vi "DCA Recalculate Values.vi"(5 "Colors":cluster{"Pass":u32, "Fail":u32, "Nop":u32}={"Pass"=6618880, "Fail"=16711680, "Nop"=16777226}, 6 "Attenuation Calculation":enum32{"Power", "Voltage"}(ring), 7 "Limit Status Ref":refnum<vi>, 8 "error in (no error)":errorcluster, 9 "Test Parameters In":T8={"Stimulus"={"Use Instrument"=FALSE, "Normalize"=FALSE, "Blank Screen"=FALSE, "Measurement Type"=enum."Diode", "Range"=enum."Auto", "Resolution"=enum."Auto"}, "Measurement"={"Topology"=enum."PI-Network", "Lock Topology"=FALSE, "ATTN Calc"=enum."Power", "Zo"=50.0}, "Limits"=[], "Normalization"={"Normalized?"=FALSE, "Rab Value"=0.0, "Rac Value"=0.0, "Rbc Value"=0.0}}, 10 "Topology":T6, 11 "Measurement Values":T7) -> (0 "error out":errorcluster, 1 "Test Parameters Out":T8={"Stimulus"={"Use Instrument"=FALSE, "Normalize"=FALSE, "Blank Screen"=FALSE, "Measurement Type"=enum."Diode", "Range"=enum."Auto", "Resolution"=enum."Auto"}, "Measurement"={"Topology"=enum."PI-Network", "Lock Topology"=FALSE, "ATTN Calc"=enum."Power", "Zo"=50.0}, "Limits"=[], "Normalization"={"Normalized?"=FALSE, "Rab Value"=0.0, "Rac Value"=0.0, "Rbc Value"=0.0}}, 2 "Passed?":bool, 3 "Measurement Values":T7, 4 "Limits and Passed?":cluster{"Limits":T1[], "Passed? Array":bool[]})   [LabVIEW 2011]
uses:
  TypeDefs/DCA Test Parameters.ctl
  TypeDefs/DCA Stimulus Parameters.ctl
  TypeDefs/DCA Measurement Cluster.ctl
  TypeDefs/DCA Topology.ctl
  TypeDefs/DCA Attenuation Calculation.ctl
  TypeDefs/DCA Limit.ctl
  TypeDefs/DCA Limit Quantity.ctl
  TypeDefs/DCA Limit Comparison.ctl
  TypeDefs/DCA Limit Operation.ctl
  Test Referential Limit.ctl
  TypeDefs/DCA Calibration State.ctl
  TypeDefs/DCA Measurement Values.ctl
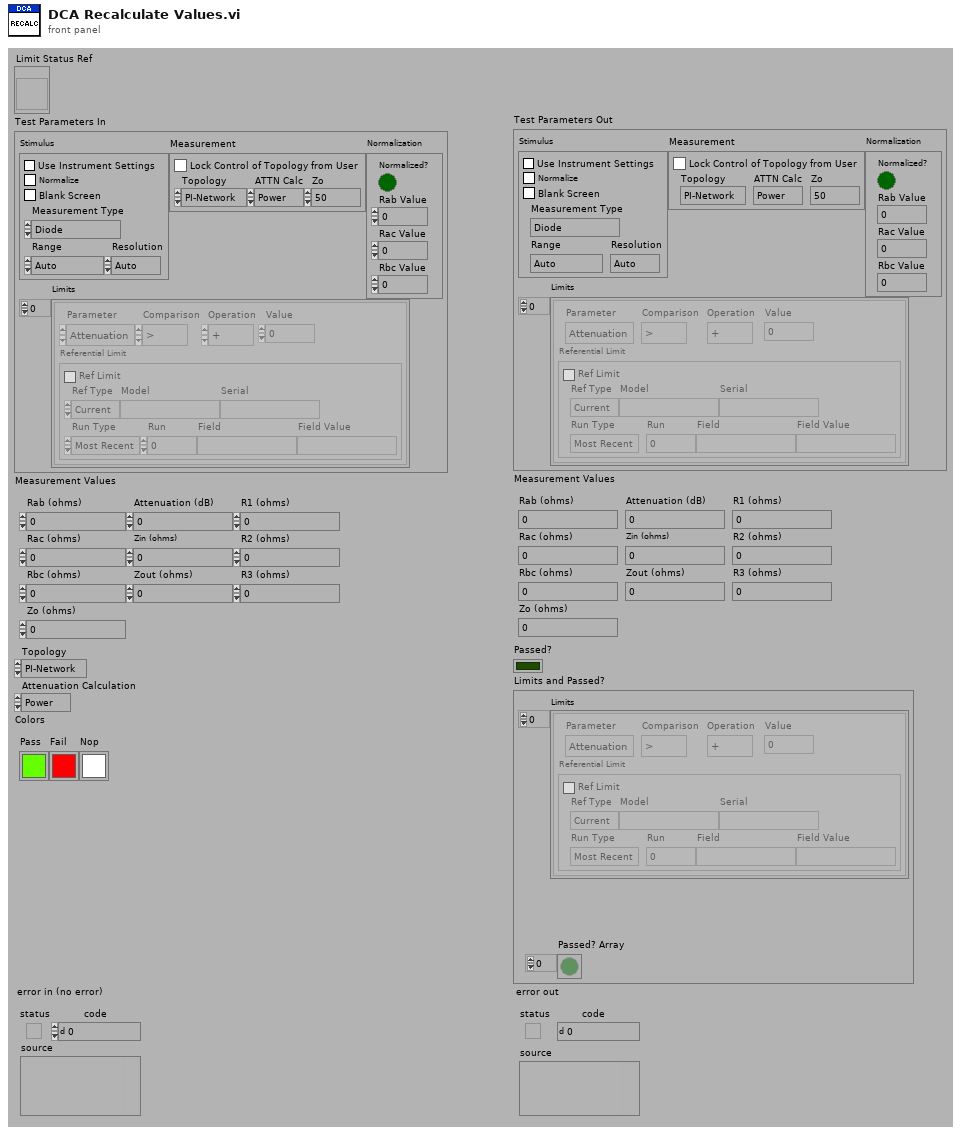
[diagram p1: front panel]
types:
  T1 = typedef "DCA Limit.ctl" = cluster{"Parameter":T2, "Comparison":T3, "Operation":T4, "Value":dbl, "Referential Limit":T5}
  T2 = typedef "DCA Limit Quantity.ctl" = enum16{"Attenuation", "Zin", "Zout", "R1", "R2", "R3", "Rab", "Rac", "Rbc"}
  T3 = typedef "DCA Limit Comparison.ctl" = enum16{">", ">=", "<", "<="}
  T4 = typedef "DCA Limit Operation.ctl" = enum16{"+", "-"}
  T5 = typedef "Test Referential Limit.ctl" = cluster{"Ref Limit":bool, "Ref Type":enum16{"Current", "Specify"}, "Model":string, "Serial":string, "Run Type":enum16{"Most Recent", "Run #", "Match Field"}, "Run":i32, "Field":string, "Field Value":string}
  T6 = typedef "DCA Topology.ctl" = enum32{"PI-Network", "T-Network"}
  T7 = typedef "DCA Measurement Values.ctl" = cluster{"Rab (ohms)":dbl, "Rac (ohms)":dbl, "Rbc (ohms)":dbl, "Zo (ohms)":dbl, "Attenuation (dB)":dbl, "Zin (ohms)":dbl, "Zout (ohms)":dbl, "R1 (ohms)":dbl, "R2 (ohms)":dbl, "R3 (ohms)":dbl}
  T8 = typedef "DCA Test Parameters.ctl" = cluster{"Stimulus":T9, "Measurement":T10, "Limits":T1[], "Normalization":T12}
  T9 = typedef "DCA Stimulus Parameters.ctl" = cluster{"Use Instrument":bool, "Normalize":bool, "Blank Screen":bool, "Measurement Type":enum16{"Voltage DC", "Voltage DC Ratio", "Voltage AC", "Current DC", "Current AC", "Resistance", "Fresistance", "Frequency", "Period", "Continuity", "Diode"}, "Range":enum16{"Auto", "Minimum", "Maximum", "100", "1,000", "10,000", "100,000", "1,000,000", "10,000,000", "100,000,000"}, "Resolution":enum16{"Auto", "4 1/2", "5 1/2", "6 1/2"}}
  T10 = typedef "DCA Measurement Cluster.ctl" = cluster{"Topology":T6, "Lock Topology":bool, "ATTN Calc":T11, "Zo":dbl}
  T11 = typedef "DCA Attenuation Calculation.ctl" = enum32{"Power", "Voltage"}
  T12 = typedef "DCA Calibration State.ctl" = cluster{"Normalized?":bool, "Rab Value":dbl, "Rac Value":dbl, "Rbc Value":dbl}
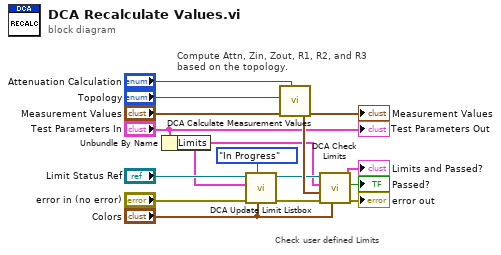
[diagram p0: block diagram]
diagram:
  # "Compute Attn, Zin, Zout, R1, R2, and R3\nbased on the topology."
  # "Check user defined Limits"
  n1 = Unbundle By Name("Test Parameters In") -> ("Limits"=w5:T1[])
  n2 = call "DCA Update Limit Listbox.vi"("Colors"="Colors", "State (Pass/Fail)"=enum16{"Reset", "In Progress", "Pass/Fail"}."In Progress", "error in (no error)"="error in (no error)", "Limits"=w5, "Limit Status Ref"="Limit Status Ref") -> ("error out"=w9:errorcluster, "Limit Status Ref Out"=w7:refnum<vi>)  [unwired: 1 in, 4 out]
  n3 = call "DCA Calculate Measurement Values.vi"("Topology"="Topology", "Measurement Values"="Measurement Values", "Attenuation Calculation"="Attenuation Calculation") -> ("Calculated Measurement Values"=w14:T7)  [unwired: 2 out]
  "Measurement Values" <- w14
  n4 = call "DCA Check Limits.vi"("Colors"="Colors", "error in (no error)"=w9, "Measurement Values"=w14, "Limits"=w5, "Limit Status Ref"=w7) -> ("error out"=→"error out":errorcluster, "Passed?"=→"Passed?":bool, "Limits and Passed?"=→"Limits and Passed?":cluster{"Limits":T1[], "Passed? Array":bool[]})  [unwired: 4 out]
  "Test Parameters Out" <- "Test Parameters In"
